vi "题目1.vi"() -> ()   [LabVIEW 2017]
uses:
  <vilib>/measure/NI_MABase.lvlib
panel:
  in  "phase":dbl caption="相位" format="%.2p"
  in  "amplitude":dbl=1.0 caption="幅值" format="%0.2p"
  in  "frequency":dbl=10.0 caption="频率" format="%0.2p"
  out "XY图":cluster{"Y":dbl[], "Y":dbl[]}(graph)
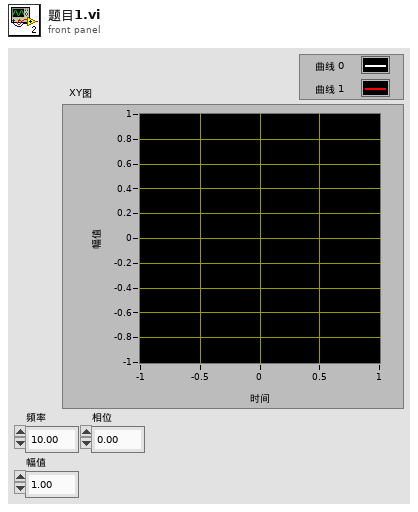
[diagram p1: front panel]
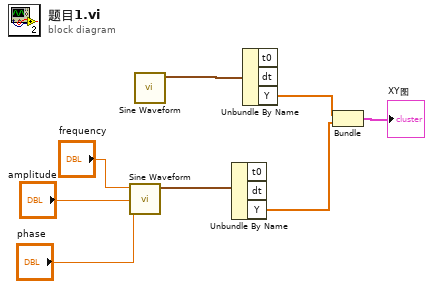
[diagram p0: block diagram]
diagram:
  n1 = call <vilib>:"Sine Waveform.vi"("phase"="phase", "amplitude"="amplitude", "frequency"="frequency") -> ("signal out"=w7:waveform(dbl))  [unwired: 7 in, 1 out]
  n2 = call <vilib>:"Sine Waveform.vi"() -> ("signal out"=w8:waveform(dbl))  [unwired: 10 in, 1 out]
  n3 = Unbundle By Name(w7) -> ("Y"=w6:dbl[])  [unwired: 2 out]
  n4 = Unbundle By Name(w8) -> ("Y"=w5:dbl[])  [unwired: 2 out]
  n5 = Bundle("Y"=w5, "Y"=w6) -> (→"XY图":cluster{"Y":dbl[], "Y":dbl[]})  [unwired: 1 in]
